vi "Get Scale.vi"(6 "Signal bits":i32=14, 7 "Number of stages":i32=6, 8 "error in (no error)":errorcluster, 9 "Range":dbl=1.0 format="%#_6eV", 10 "Channel":i32, 11 "RP Instrument in":refnum<class "RP Instrument.lvclass">) -> (0 "error out":errorcluster, 1 "slope":dbl, 2 "y intersept":dbl, 3 "RP Instrument out":refnum<class "RP Instrument.lvclass">, 4 "RP EEPROM Calibration":T1 {"magic" format="%x"})   [LabVIEW 2019, in "RP Instrument.lvclass"]
uses:
  RP Instrument.lvclass
  RP EEPROM Calibration.ctl
  RP Instrument.lvclass/RP Instrument.ctl
  RP Communicator/RP Communicator.lvclass/RP Communicator.ctl
  RP Communicator/Read RP EEPROM Calibration.vi
  RP Communicator/RP Communicator.lvclass
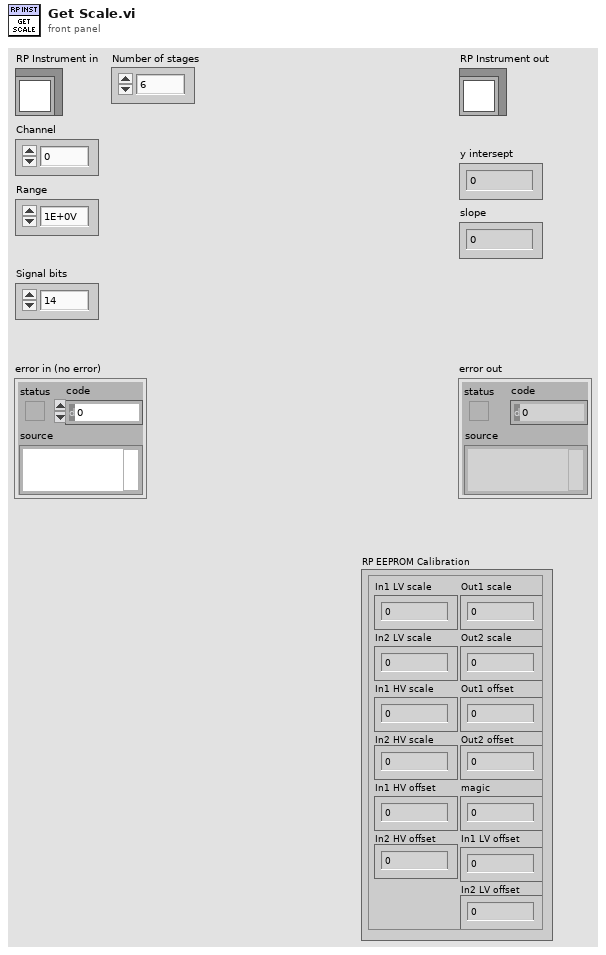
[diagram p1: front panel]
types:
  T1 = typedef "RP EEPROM Calibration.ctl" = cluster{"In1 LV scale":u32, "In2 LV scale":u32, "In1 HV scale":u32, "In2 HV scale":u32, "In1 HV offset":i32, "In2 HV offset":i32, "Out1 scale":u32, "Out2 scale":u32, "Out1 offset":i32, "Out2 offset":i32, "magic":u32, "In1 LV offset":i32, "In2 LV offset":i32}
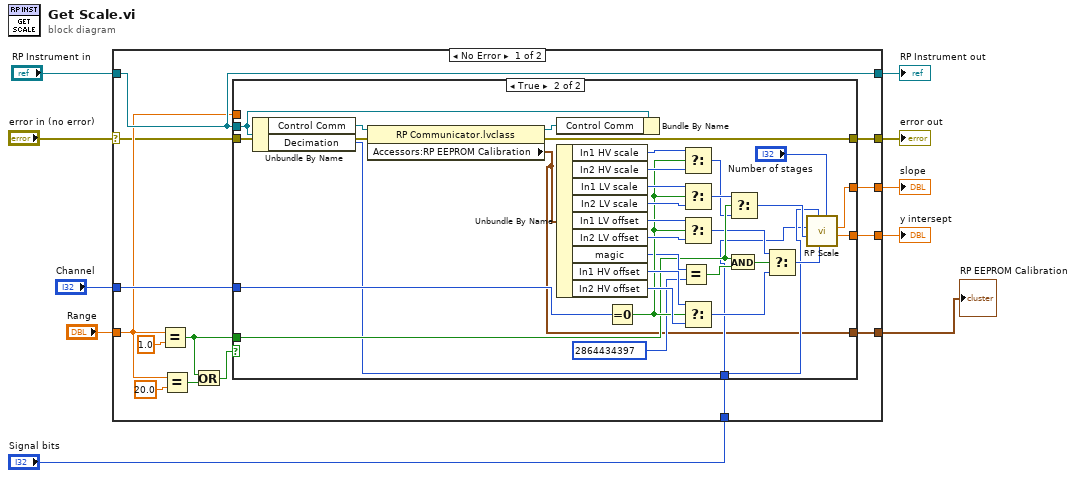
[diagram p0: block diagram]
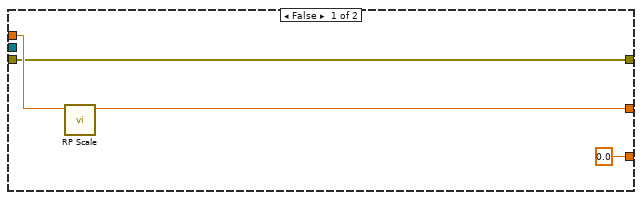
[diagram p2: hidden frame]
diagram:
  n1 = case shown="No Error" "error in (no error)" {
    selector: "error in (no error)" -> [w15 w62]
    tunnel: [w14 w62] -> w9
    tunnel: [w21 w61] -> w7
    tunnel: "RP Instrument in" -> [w21 w61]
    tunnel: "Range" -> [w17 _]
    tunnel: "Channel" -> [w20 _]
    tunnel: [w18 _] -> w4
    tunnel: [w16 _] -> w3
    tunnel: "Signal bits" -> [w12 _]
    tunnel: [w11 _] -> w1
    frame No Error {
      n2 = Equal?(x=w17, y=1.0) -> (x = y?=w13:bool)
      n3 = Equal?(x=w17, y=20.0) -> (x = y?=w19:bool)
      n4 = Or(x=w13, y=w19) -> (x .or. y?=w22:bool)
      n5 = case shown="True" w22 {
        tunnel: w21 -> [_ w44]
        tunnel: w20 -> [_ w57]
        tunnel: w13 -> [_ w46]
        tunnel: [0.0 w37] -> w18
        tunnel: w17 -> [w27 _]
        tunnel: [w26 w38] -> w16
        tunnel: w15 -> [w25 w42]
        tunnel: [w25 w41] -> w14
        tunnel: w12 -> [_ w30]
        tunnel: [_ w29] -> w11
        frame False {
          n6 = call "RP Scale.vi"("Range"=w27) -> ("Slope"=w26:dbl)  [unwired: 8 in, 2 out]
        }
        frame True {
          n7 = Unbundle By Name(w44) -> ("Control Comm"=w60:refnum<class "RP Communicator.lvclass">, "Decimation"=w32:u32)
          n8 = property class="RP Communicator.lvclass"(reference=w60, error in=w42) -> (reference out=w43:refnum<class "RP Communicator.lvclass">, error out=w41:errorcluster, "Accessors:RP EEPROM Calibration"=w29:T1)
          n9 = Bundle By Name(cluster=w44, "Control Comm"=w43) -> ()  [unwired: 1 out]
          n10 = Unbundle By Name(w29) -> ("In1 HV scale"=w59:u32, "In2 HV scale"=w58:u32, "In1 LV scale"=w56:u32, "In2 LV scale"=w55:u32, "In1 LV offset"=w54:i32, "In2 LV offset"=w53:i32, "magic"=w49:u32, "In1 HV offset"=w52:i32, "In2 HV offset"=w51:i32)
          n11 = Equal To 0?(x=w57) -> (x = 0?=w50:bool)
          n12 = Equal?(x=w49, y=u32 2864434397) -> (x = y?=w47:bool)
          n13 = Select(t=w59, s=w50, f=w58) -> (s? t:f=w33:u32)
          n14 = Select(t=w56, s=w50, f=w55) -> (s? t:f=w34:u32)
          n15 = Select(t=w54, s=w50, f=w53) -> (s? t:f=w36:i32)
          n16 = Select(t=w52, s=w50, f=w51) -> (s? t:f=w35:i32)
          n17 = And(x=w46, y=w47) -> (x .and. y?=w45:bool)
          n18 = Select(t=w34, s=w46, f=w33) -> (s? t:f=w40:u32)
          n19 = Select(t=w36, s=w45, f=w35) -> (s? t:f=w39:i32)
          n20 = call "RP Scale.vi"("Number of stages"="Number of stages", "EEPROM offset"=w39, "Decimation"=w32, "EEPROM range"=w40, "Signal bits"=w30) -> ("y intersept"=w37:dbl, "Calibrated slope"=w38:dbl)  [unwired: 4 in, 1 out]
        }
      }
    }
    frame Error {
    }
  }
  "error out" <- w9
  "RP Instrument out" <- w7
  "slope" <- w3
  "y intersept" <- w4
  "RP EEPROM Calibration" <- w1
